vi "send outputs to fpga.vi"(7 "outputs":T2[](array[typedef]), 8 "error in":errorcluster, 9 "command list":u32[](array[numeric]), 10 "data table in in":T1, 11 "FPGA in":T5) -> (0 "error out":errorcluster, 3 "data table out":T1)   [LabVIEW 2013, in "Profibus Module runtime.lvclass"]
uses:
  Profibus Module runtime.lvclass
  dynamic profibus/fpga reference.ctl
  profibus slave configuration.ctl
  profibus mapping configuration.ctl
  <vilib>/NI/Tag Bus/tag/Data Type.ctl
  <vilib>/NI/Tag Bus/table/data table.ctl
  dynamic profibus/dynamic profibus.lvlib
  <vilib>/NI/Tag Bus/tag/tag descriptor.lvclass
  <vilib>/NI/Tag Bus/table/data table.lvlib
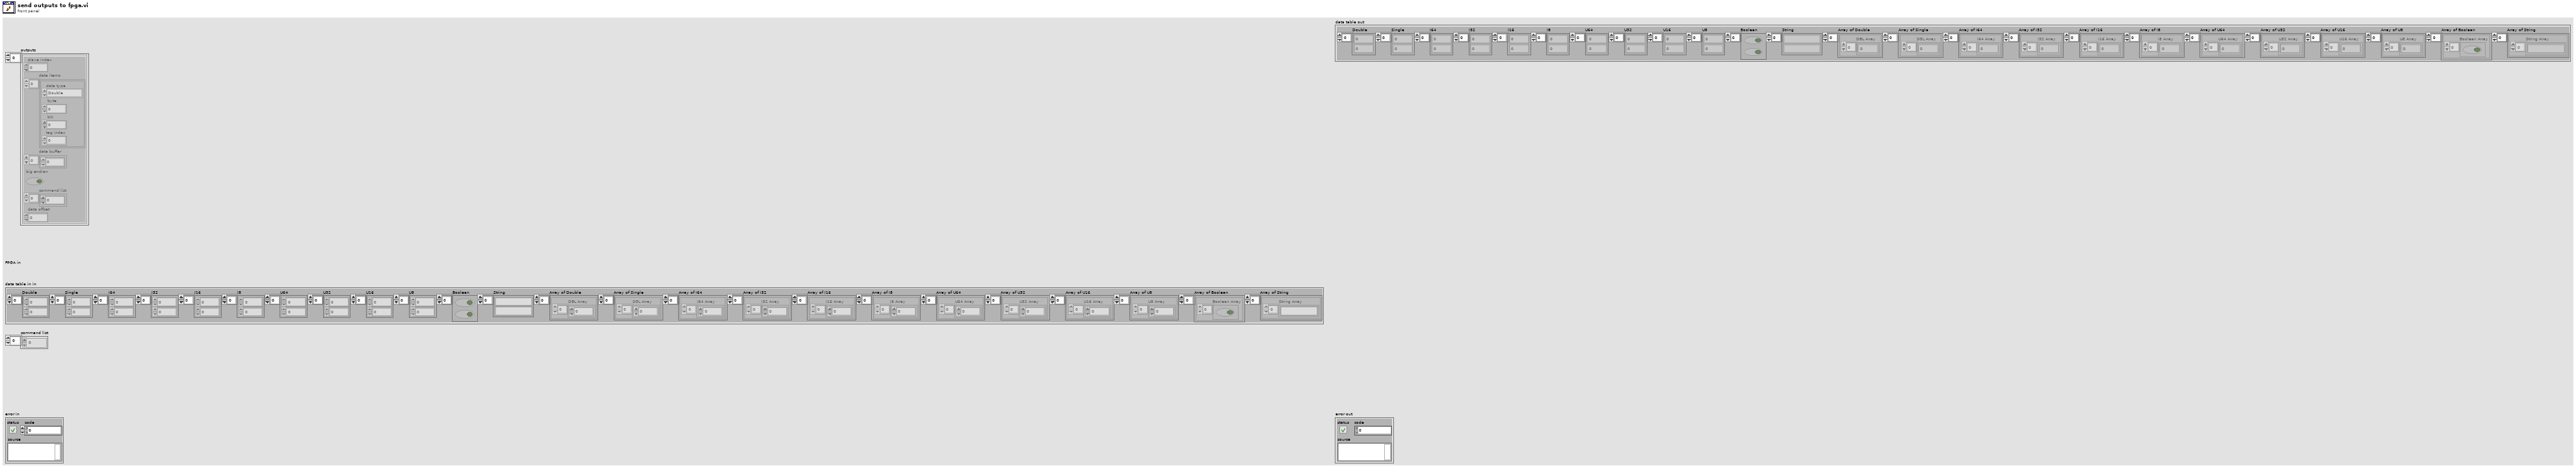
[diagram p1: front panel]
types:
  T1 = typedef "tag bus.lvlib/data table.lvlib/data table.ctl" = cluster{"Double":dbl[], "Single":sgl[], "I64":i64[], "I32":i32[], "I16":i16[], "I8":i8[], "U64":u64[], "U32":u32[], "U16":u16[], "U8":u8[], "Boolean":bool[], "String":string[], "Array of Double":cluster{"DBL Array":dbl[]}[], "Array of Single":cluster{"SGL Array":sgl[]}[], "Array of I64":cluster{"I64 Array":i64[]}[], "Array of I32":cluster{"I32 Array":i32[]}[], "Array of I16":cluster{"I16 Array":i16[]}[], "Array of I8":cluster{"I8 Array":i8[]}[], "Array of U64":cluster{"U64 Array":u64[]}[], "Array of U32":cluster{"U32 Array":u32[]}[], "Array of U16":cluster{"U16 Array":u16[]}[], "Array of U8":cluster{"U8 Array":u8[]}[], "Array of Boolean":cluster{"Boolean Array":bool[]}[], "Array of String":cluster{"String Array":string[]}[]}
  T2 = typedef "Profibus Module runtime.lvclass/profibus slave configuration.ctl" = cluster{"slave index":i8, "data items":T3[], "data buffer":u8[], "big endian":bool, "command list":u32[], "data offset":u8}
  T3 = typedef "Profibus Module runtime.lvclass/profibus mapping configuration.ctl" = cluster{"data type":T4, " byte":i32, " bit":i32, "tag index":i32}
  T4 = typedef "tag bus.lvlib/tag descriptor.lvclass/Data Type.ctl" = enum16{"Double", "Single", "I64", "I32", "I16", "I8", "U64", "U32", "U16", "U8", "Boolean", "String", "Array of Double", "Array of Single", "Array of I64", "Array of I32", "Array of I16", "Array of I8", "Array of U64", "Array of U32", "Array of U16", "Array of U8", "Array of Boolean", "Array of String"}
  T5 = typedef "dynamic profibus.lvlib/fpga reference.ctl" = refnum<k20>
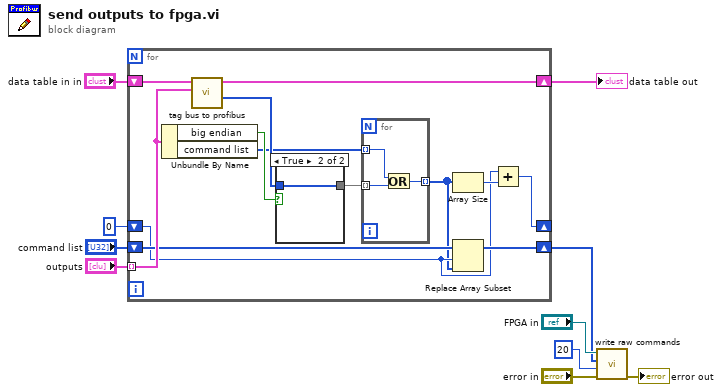
[diagram p0: block diagram]
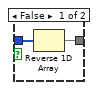
[diagram p2: hidden frame]
diagram:
  n1 = for {
    shift-right: [w22] -> w7
    shift-left: "data table in in" -> [w23]
    tunnel: "outputs" -> [w21] mode=indexing
    shift-right: [w15] -> w1
    shift-left: "command list" -> [w16]
    shift-right: [w17] -> _
    shift-left: 0 -> [w14]
    n2 = Unbundle By Name(w21) -> ("big endian"=w20:bool, "command list"=w12:u32[])
    n3 = call "tag bus to profibus.vi"("slave configuration"=w21, "data table in in"=w23) -> ("Data"=w19:u8[], "data table out"=w22:T1)  [unwired: 7 in, 1 out]
    n4 = case shown="True" w20 {
      tunnel: [w27 w29] -> w13
      tunnel: w19 -> [w28 w29]
      frame False {
        n5 = Reverse 1D Array(array=w28) -> (reversed array=w27:u8[])
      }
      frame True {
      }
    }
    n6 = for {
      tunnel: w13 -> [w26] mode=indexing
      tunnel: w12 -> [w25] mode=indexing
      tunnel: [w24] -> w11 mode=indexing
      n7 = Or(x=w25, y=w26) -> (x .or. y?=w24:u32)
    }
    n8 = Array Size(array=w11) -> (size(s)=w18:i32)
    n9 = Replace Array Subset(array=w16, new element=w11, index=w14) -> (w15:u32[])
    n10 = Add(x=w14, y=w18) -> (x+y=w17:i32)
  }
  "data table out" <- w7
  n11 = call "write raw commands.vi"("error in"="error in", "Timeout (ms)"=20, "Data"=w1, "profibus reference"="FPGA in") -> ("error out"=→"error out":errorcluster)  [unwired: 5 in, 2 out]
